vi "Adjust Cursor Y Position to Maintain Label Placement.vi"(10 "Refnums for Resizing and Alignment":T1, 11 "Display State In":T2={"Graph Visible Items"={"Plot Legend"=FALSE, "Scale Legend"=FALSE, "Graph Palette"=FALSE, "Cursor Legend"=FALSE, "X Scrollbar"=FALSE}, "View Table"=FALSE, "Table Visible Items"={"Vertical Scrollbar"=FALSE, "Horizontal Scrollbar"=FALSE, "Row Headers"=FALSE, "Column Headers"=FALSE, "Vertical Lines"=FALSE, "Horizontal Lines"=FALSE}, "Header Font"={"Font Name"="", "Size"=0, "Bold"=FALSE, "Italic"=FALSE, "Underline"=FALSE, "Strikeout"=FALSE, "Color"=0}, "Cell Font"={"Font Name"="", "Size"=0, "Bold"=FALSE, "Italic"=FALSE, "Underline"=FALSE, "Strikeout"=FALSE, "Color"=0}, "Description and Tip..."={"Description"="", "Tip"=""}, "Moveable Splitter Position"=0, "Measurement Cursor Configuration"={"XY"={"enable XY"=FALSE, "Position (X)"=[], "Type"=enum."Absolute", "Y reference"=0.0, "color"=0}, "band"={"enable band"=FALSE, "B1"=0.0, "B2"=0.0, "Fixed bandwidth (B2-B1)"=0.0, "B1 color"=0, "B2 color"=0}, "harmonic"={"enable harmonics"=FALSE, "X reference (1X)"=0.0, "Maximum"=0, "Subset"=enum."All", "1X color"=0, "MX color"=0}, "sideband"={"enable sideband"=FALSE, "X center (C)"=0.0, "Sidebands"=0, "X spacing (s)"=0.0, "Center color"=0, "Sideband color"=0}}, "Cursors"={"List"=[], "Tags"=[]}, "X Increment"=0.0, "X Scale"={"Label Visible"=FALSE, "Label Text"="", "Mapping Mode"=0, "Format String"=""}, "Y Scale"={"Label Visible"=FALSE, "Label Text"="", "Mapping Mode"=0, "Format String"=""}, "Colors"={"background"=16777215, "major grid"=8355711, "minor grid"=12632256, "font"=0}, "desired spectrum view"={"scaling"={"linear/dB"=enum."no change", "dB reference"=0.0, "power/magnitude"=enum."no change", "view"=enum."no change"}, "spectral density"=enum."no change"}, "Plot Color Wheel"=[3381759, 32768, 982784, 4375295, 13827953, 13457919, 16757522, 4343295, 16728758, 12095254], "Plots"=[], "registered user events"=variant, "Lock 1X to Peak"=FALSE} caption="State" {"Y Scale"."Mapping Mode" items=["Linear", "Logarithmic", "dB"]; "X Scale"."Mapping Mode" items=["Linear", "Logarithmic"]}) -> (3 "Display State Out":T2={"Graph Visible Items"={"Plot Legend"=FALSE, "Scale Legend"=FALSE, "Graph Palette"=FALSE, "Cursor Legend"=FALSE, "X Scrollbar"=FALSE}, "View Table"=FALSE, "Table Visible Items"={"Vertical Scrollbar"=FALSE, "Horizontal Scrollbar"=FALSE, "Row Headers"=FALSE, "Column Headers"=FALSE, "Vertical Lines"=FALSE, "Horizontal Lines"=FALSE}, "Header Font"={"Font Name"="", "Size"=0, "Bold"=FALSE, "Italic"=FALSE, "Underline"=FALSE, "Strikeout"=FALSE, "Color"=0}, "Cell Font"={"Font Name"="", "Size"=0, "Bold"=FALSE, "Italic"=FALSE, "Underline"=FALSE, "Strikeout"=FALSE, "Color"=0}, "Description and Tip..."={"Description"="", "Tip"=""}, "Moveable Splitter Position"=0, "Measurement Cursor Configuration"={"XY"={"enable XY"=FALSE, "Position (X)"=[], "Type"=enum."Absolute", "Y reference"=0.0, "color"=0}, "band"={"enable band"=FALSE, "B1"=0.0, "B2"=0.0, "Fixed bandwidth (B2-B1)"=0.0, "B1 color"=0, "B2 color"=0}, "harmonic"={"enable harmonics"=FALSE, "X reference (1X)"=0.0, "Maximum"=0, "Subset"=enum."All", "1X color"=0, "MX color"=0}, "sideband"={"enable sideband"=FALSE, "X center (C)"=0.0, "Sidebands"=0, "X spacing (s)"=0.0, "Center color"=0, "Sideband color"=0}}, "Cursors"={"List"=[], "Tags"=[]}, "X Increment"=0.0, "X Scale"={"Label Visible"=FALSE, "Label Text"="", "Mapping Mode"=0, "Format String"=""}, "Y Scale"={"Label Visible"=FALSE, "Label Text"="", "Mapping Mode"=0, "Format String"=""}, "Colors"={"background"=16777215, "major grid"=8355711, "minor grid"=12632256, "font"=0}, "desired spectrum view"={"scaling"={"linear/dB"=enum."no change", "dB reference"=0.0, "power/magnitude"=enum."no change", "view"=enum."no change"}, "spectral density"=enum."no change"}, "Plot Color Wheel"=[3381759, 32768, 982784, 4375295, 13827953, 13457919, 16757522, 4343295, 16728758, 12095254], "Plots"=[], "registered user events"=variant, "Lock 1X to Peak"=FALSE} caption="State" {"Y Scale"."Mapping Mode" items=["Linear", "Logarithmic", "dB"]; "X Scale"."Mapping Mode" items=["Linear", "Logarithmic"]})   [LabVIEW 2017, in "Octave with Cursors.xctl"]
doc: "Use whenever y-scale changes to keep cursor positions and labels at the desired margin in the plot area"
uses:
  <vilib>/addons/_XControls/Octave with Cursors/Octave with Cursors.xctl
  <vilib>/addons/_XControls/Octave with Cursors/Controls/State.ctl
  <vilib>/Utility/miscctls.llb/LVFontTypeDef.ctl
  <vilib>/addons/_XControls/Octave with Cursors/Controls/Measurement Cursor Configuration.ctl
  <vilib>/addons/_XControls/Octave with Cursors/Controls/Refnums Typedef.ctl
  <vilib>/addons/Sound and Vibration/svt_Controls/subVIs/Multiplot Octave Graph.ctl
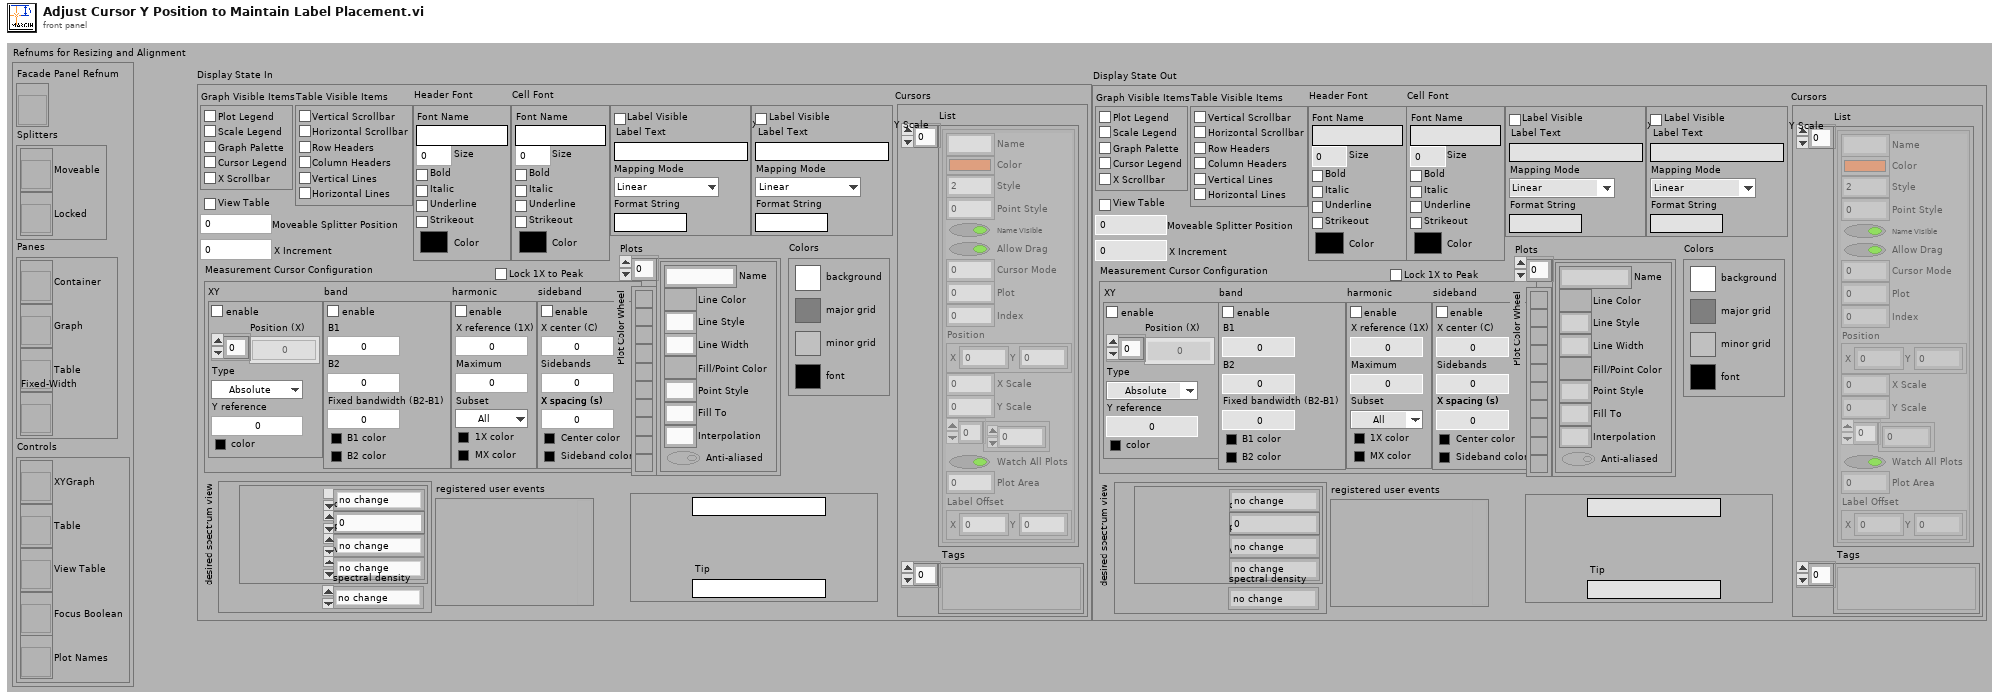
[diagram p1: front panel]
types:
  T1 = typedef "Octave with Cursors.xctl/Refnums Typedef.ctl" = cluster{"Facade Panel Refnum":refnum<vi>, "Splitters":cluster{"Moveable":refnum<vi>, "Locked":refnum<vi>}, "Panes":cluster{"Container":refnum<vi>, "Graph":refnum<vi>, "Table":refnum<vi>, "Fixed-Width":refnum<vi>}, "Controls":cluster{"XYGraph":refnum<vi>, "Table":refnum<vi>, "View Table":refnum<vi>, "Focus Boolean":refnum<vi>, "Plot Names":refnum<vi>}}
  T2 = typedef "Octave with Cursors.xctl/State.ctl" = cluster{"Graph Visible Items":cluster{"Plot Legend":bool, "Scale Legend":bool, "Graph Palette":bool, "Cursor Legend":bool, "X Scrollbar":bool}, "View Table":bool, "Table Visible Items":cluster{"Vertical Scrollbar":bool, "Horizontal Scrollbar":bool, "Row Headers":bool, "Column Headers":bool, "Vertical Lines":bool, "Horizontal Lines":bool}, "Header Font":T3, "Cell Font":T3, "Description and Tip...":cluster{"Description":string, "Tip":string}, "Moveable Splitter Position":i32, "Measurement Cursor Configuration":T4, "Cursors":cluster{"List":cluster{"Name":string, "Color":u32, "Style":i32, "Point Style":u8, "Name Visible":bool, "Allow Drag":bool, "Cursor Mode":u32, "Plot":i32, "Index":i32, "Position":cluster{"X":dbl, "Y":dbl}, "X Scale":u32, "Y Scale":u32, "Watch Plots":i32[], "Watch All Plots":bool, "Plot Area":i32, "Label Offset":cluster{"X":dbl, "Y":dbl}}[], "Tags":variant[]}, "X Increment":dbl, "X Scale":cluster{"Label Visible":bool, "Label Text":string, "Mapping Mode":u8, "Format String":string}, "Y Scale":cluster{"Label Visible":bool, "Label Text":string, "Mapping Mode":u8, "Format String":string}, "Colors":cluster{"background":u32, "major grid":u32, "minor grid":u32, "font":u32}, "desired spectrum view":cluster{"scaling":cluster{"linear/dB":enum16{"no change", "linear", "dB"}, "dB reference":dbl, "power/magnitude":enum16{"no change", "power", "magnitude"}, "view":enum16{"no change", "rms", "peak", "peak-peak"}}, "spectral density":enum16{"no change", "spectrum", "spectral density"}}, "Plot Color Wheel":u32[], "Plots":cluster{"Name":string, "Line Color":u32, "Line Style":u8, "Line Width":u8, "Fill/Point Color":u32, "Point Style":u8, "Fill To":i16, "Interpolation":u8, "Anti-aliased":bool}[], "registered user events":variant, "Lock 1X to Peak":bool}
  T3 = typedef "LVFontTypeDef.ctl" = cluster{"Font Name":string, "Size":u16, "Bold":bool, "Italic":bool, "Underline":bool, "Strikeout":bool, "Color":u32}
  T4 = typedef "Octave with Cursors.xctl/Measurement Cursor Configuration.ctl" = cluster{"XY":cluster{"enable XY":bool, "Position (X)":dbl[], "Type":enum16{"Absolute", "Relative"}, "Y reference":dbl, "color":u32}, "band":cluster{"enable band":bool, "B1":dbl, "B2":dbl, "Fixed bandwidth (B2-B1)":dbl, "B1 color":u32, "B2 color":u32}, "harmonic":cluster{"enable harmonics":bool, "X reference (1X)":dbl, "Maximum":i32, "Subset":enum16{"All", "Even", "Odd"}, "1X color":u32, "MX color":u32}, "sideband":cluster{"enable sideband":bool, "X center (C)":dbl, "Sidebands":i32, "X spacing (s)":dbl, "Center color":u32, "Sideband color":u32}}
  T5 = cluster{"Name":string, "Color":u32, "Style":i32, "Point Style":u8, "Name Visible":bool, "Allow Drag":bool, "Cursor Mode":u32, "Plot":i32, "Index":i32, "Position":cluster{"X":dbl, "Y":dbl}, "X Scale":u32, "Y Scale":u32, "Watch Plots":i32[], "Watch All Plots":bool, "Plot Area":i32, "Label Offset":cluster{"X":dbl, "Y":dbl}}[]
  T6 = cluster{"Name":string, "Color":u32, "Style":i32, "Point Style":u8, "Name Visible":bool, "Allow Drag":bool, "Cursor Mode":u32, "Plot":i32, "Index":i32, "Position":cluster{"X":dbl, "Y":dbl}, "X Scale":u32, "Y Scale":u32, "Watch Plots":i32[], "Watch All Plots":bool, "Plot Area":i32, "Label Offset":cluster{"X":dbl, "Y":dbl}}
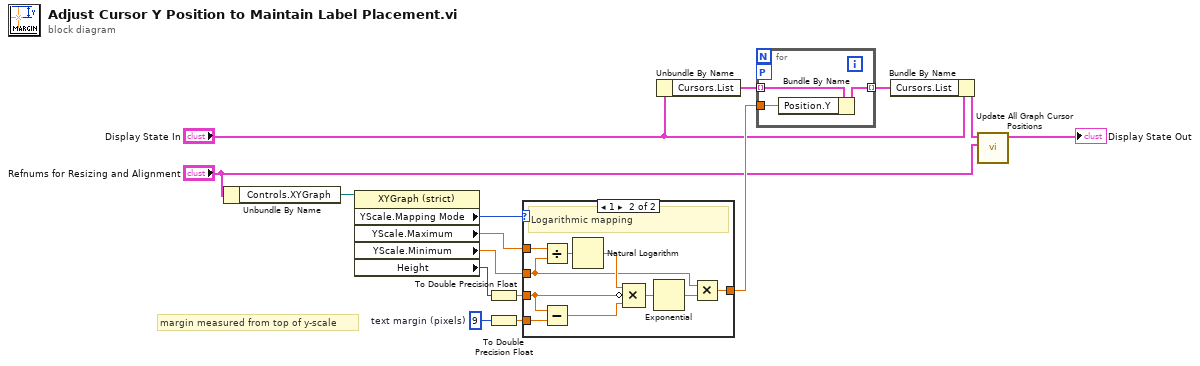
[diagram p0: block diagram]
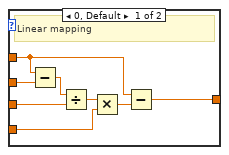
[diagram p2: hidden frame]
diagram:
  w12 = 9  # text margin (pixels)
  # "margin measured from top of y-scale"
  n1 = Unbundle By Name("Refnums for Resizing and Alignment") -> ("Controls.XYGraph"=w15:refnum<vi>)
  n2 = property class="XYGraph (strict)"(reference=w15) -> ("YScale.Mapping Mode"=w8:u8, "YScale.Maximum"=w9:dbl, "YScale.Minimum"=w10:dbl, "Height"=w11:u32)  [unwired: 1 in, 2 out]
  n3 = To Double Precision Float(number=w11) -> (double precision float=w13:dbl)
  n4 = To Double Precision Float(number=w12) -> (double precision float=w14:dbl)
  n5 = case shown="1" w8 {
    tunnel: w9 -> [w18 w30]
    tunnel: w10 -> [w20 w24]
    tunnel: w13 -> [w19 w32]
    tunnel: [w17 w25] -> w7
    tunnel: w14 -> [w16 w33]
    frame 0, Default {
      # "Linear mapping"
      n6 = Subtract(x=w18, y=w20) -> (x-y=w21:dbl)
      n7 = Divide(x=w21, y=w19) -> (x/y=w22:dbl)
      n8 = Multiply(x=w22, y=w16) -> (x*y=w23:dbl)
      n9 = Subtract(x=w18, y=w23) -> (x-y=w17:dbl)
    }
    frame 1 {
      # "Logarithmic mapping"
      n10 = Divide(x=w30, y=w24) -> (x/y=w29:dbl)
      n11 = Subtract(x=w32, y=w33) -> (x-y=w31:dbl)
      n12 = Natural Logarithm(1:w29) -> (0:w28:dbl)
      n13 = Compound Arithmetic op=MULTIPLY(w28, invert w32, w31) -> (w27:dbl)
      n14 = Exponential(1:w27) -> (0:w26:dbl)
      n15 = Multiply(x=w24, y=w26) -> (x*y=w25:dbl)
    }
  }
  n16 = Unbundle By Name("Display State In") -> ("Cursors.List"=w6:T5)
  n17 = for {
    tunnel: w7 -> [w34]
    tunnel: w6 -> [w36] mode=indexing
    tunnel: [w35] -> w5 mode=indexing
    workers-P: _ -> [_]
    n18 = Bundle By Name(cluster=w36, "Position.Y"=w34) -> (w35:T6)
  }
  n19 = Bundle By Name(cluster="Display State In", "Cursors.List"=w5) -> (w4:T2)
  n20 = call <vilib>:"Update All Graph Cursor Positions.vi"("Refnums for Resizing and Alignment"="Refnums for Resizing and Alignment", "Display State In"=w4) -> ("Display State Out"=→"Display State Out":T2)  [unwired: 9 in]
